vi "ex_4_11.vi"() -> ()   [LabVIEW 2020]
uses:
  <vilib>/regexp/Match Regular Expression.xnode
panel:
  out "valid?":bool=TRUE
  in  "String":string
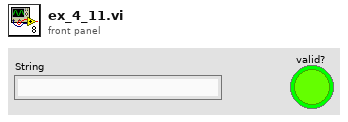
[diagram p1: front panel]
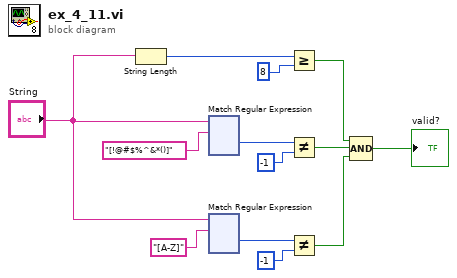
[diagram p0: block diagram]
diagram:
  n1 = String Length(string="String") -> (length=w5:i32)
  n2 = xnode "Match Regular Expression"("input string"="String", "regular expression"="[!@#$%^&*()]") -> ("offset past match"=w7:i32)  [unwired: 4 in, 4 out]
  n3 = xnode "Match Regular Expression"("input string"="String", "regular expression"="[A-Z]") -> ("offset past match"=w11:i32)  [unwired: 4 in, 4 out]
  n4 = Greater Or Equal?(x=w5, y=8) -> (x >= y?=w4:bool)
  n5 = Not Equal?(x=w7, y=-1) -> (x != y?=w3:bool)
  n6 = Not Equal?(x=w11, y=-1) -> (x != y?=w2:bool)
  n7 = Compound Arithmetic op=AND(w4, w3, w2) -> (→"valid?":bool)
